vi "getAdditionalDataFromXML.vi"(8 "error in (no error)":errorcluster, 10 "Xml":refnum<class "xmlNode.lvclass">, 11 "RampEvent in":refnum<class "RampEvent.lvclass">) -> (0 "error out":errorcluster, 2 "Xml out":refnum<class "xmlNode.lvclass">, 3 "RampEvent out":refnum<class "RampEvent.lvclass">)   [LabVIEW 2011, in "Tools.lvlib" / "Scripting.lvlib" / "RampEvent.lvclass"]
uses:
  RampEvent.lvclass
  xmlNode/xmlNode.lvclass
  RampEvent.lvclass/RampEvent.ctl
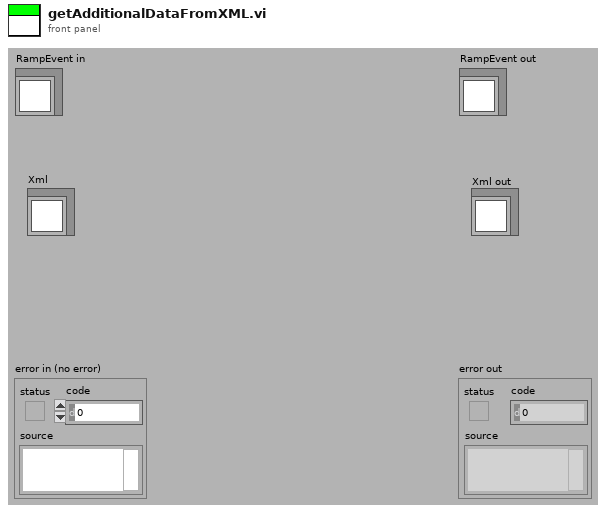
[diagram p1: front panel]
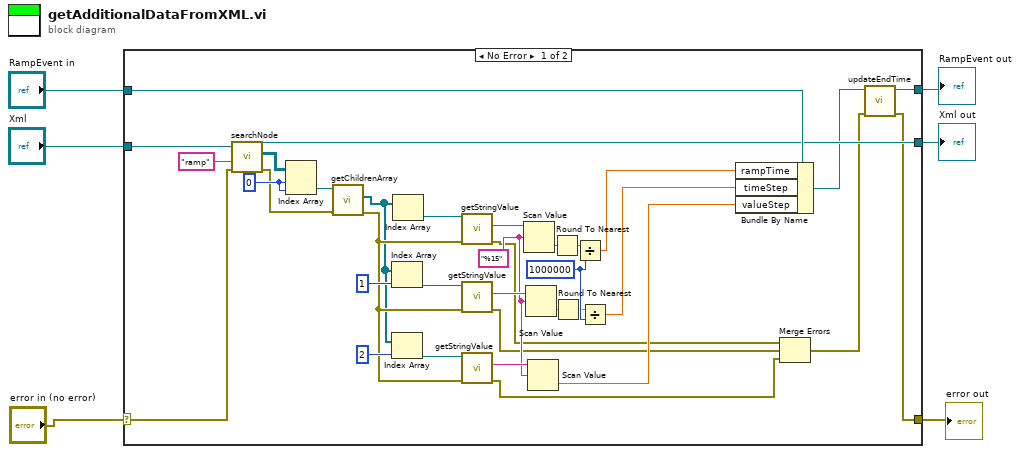
[diagram p0: block diagram]
diagram:
  n1 = case shown="No Error" "error in (no error)" {
    selector: "error in (no error)" -> [w33 w42]
    tunnel: [w9 w42] -> w5
    tunnel: "RampEvent in" -> [w20 w44]
    tunnel: [w11 w44] -> w3
    tunnel: "Xml" -> [w34 w43]
    tunnel: [w19 w43] -> w1
    frame No Error {
      w23 = 1000000
      w17 = "%15"
      w39 = 0
      n2 = call-dynamic "searchNode.vi"("error in (no error)"=w33, "searchElementName"="ramp", "xmlNode in"=w34) -> ("error out"=w37:errorcluster, "arrayXmlNodes"=w40:refnum<class "xmlNode.lvclass">[][], "xmlNode out"=w19:refnum<class "xmlNode.lvclass">)  [unwired: 6 in]
      n3 = Index Array(array=w40, index (row)=w39, index (col)=w39) -> (element=w38:refnum<class "xmlNode.lvclass">)
      n4 = call-dynamic "getChildrenArray.vi"("error in (no error)"=w37, "xmlNode.lvclass in"=w38) -> ("error out"=w29:errorcluster, "Children"=w28:refnum<class "xmlNode.lvclass">[])  [unwired: 7 in, 1 out]
      n5 = Index Array(array=w28, index=1) -> (element=w35:refnum<class "xmlNode.lvclass">)
      n6 = Index Array(array=w28, index=2) -> (element=w31:refnum<class "xmlNode.lvclass">)
      n7 = Index Array(array=w28) -> (element=w36:refnum<class "xmlNode.lvclass">)  [unwired: 1 in]
      n8 = call-dynamic "getStringValue.vi"("error in (no error)"=w29, "xmlNode.lvclass in"=w36) -> ("error out"=w15:errorcluster, "stringValue"=w27:string)  [unwired: 7 in, 1 out]
      n9 = call-dynamic "getStringValue.vi"("error in (no error)"=w29, "xmlNode.lvclass in"=w35) -> ("error out"=w14:errorcluster, "stringValue"=w26:string)  [unwired: 7 in, 1 out]
      n10 = call-dynamic "getStringValue.vi"("error in (no error)"=w29, "xmlNode.lvclass in"=w31) -> ("error out"=w13:errorcluster, "stringValue"=w18:string)  [unwired: 7 in, 1 out]
      n11 = Scan Value(string=w27, format string=w17) -> (value=w25:dbl)  [unwired: 1 in, 1 out]
      n12 = Scan Value(string=w26, format string=w17) -> (value=w24:dbl)  [unwired: 1 in, 1 out]
      n13 = Scan Value(string=w18, format string=w17) -> (value=w16:dbl)  [unwired: 1 in, 1 out]
      n14 = Round To Nearest(number=w25) -> (nearest integer value=w8:dbl)
      n15 = Round To Nearest(number=w24) -> (nearest integer value=w7:dbl)
      n16 = Divide(x=w8, y=w23) -> (x/y=w22:dbl)
      n17 = Divide(x=w7, y=w23) -> (x/y=w21:dbl)
      n18 = Bundle By Name(cluster=w20, "rampTime"=w22, "timeStep"=w21, "valueStep"=w16) -> (w12:refnum<class "RampEvent.lvclass">)
      n19 = Merge Errors(w15, w14, w13) -> (w10:errorcluster)
      n20 = call-dynamic "updateEndTime.vi"("error in (no error)"=w10, "RampEvent in"=w12) -> ("error out"=w9:errorcluster, "RampEvent out"=w11:refnum<class "RampEvent.lvclass">)  [unwired: 8 in]
    }
    frame Error {
    }
  }
  "error out" <- w5
  "RampEvent out" <- w3
  "Xml out" <- w1
